vi "IMU.vi"(8 "error in (no error)":errorcluster, 11 "VISA Refnum in":refnum<visa-resource-name>) -> (0 "error out":errorcluster, 1 "Waveform Chart":cluster{"Yaw":dbl, "Pitch":dbl, "Roll":dbl}(graph), 2 "IMU Text":string, 3 "VISA Refnum out":refnum<visa-resource-name>, 5 "IMU Data Cluster":T1)   [LabVIEW 2016]
uses:
  Project Custom Controls/IMU Data Cluster.ctl
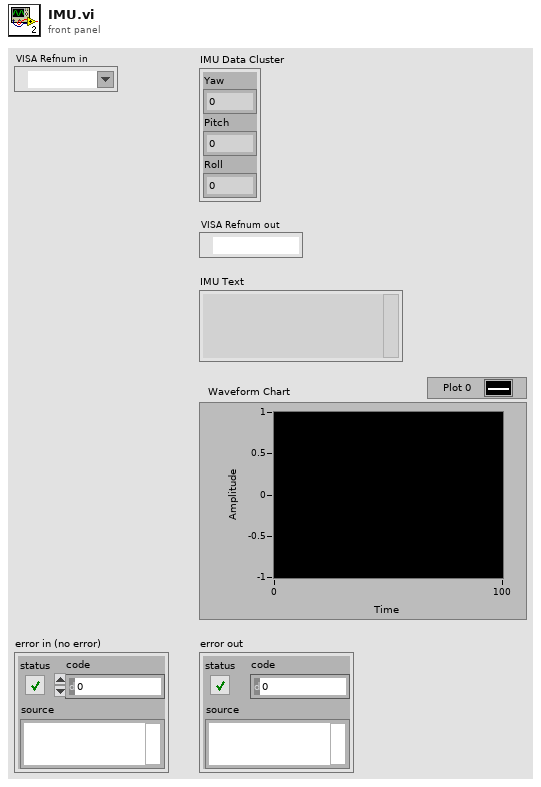
[diagram p1: front panel]
types:
  T1 = typedef "IMU Data Cluster.ctl" = cluster{"Yaw":dbl, "Pitch":dbl, "Roll":dbl}
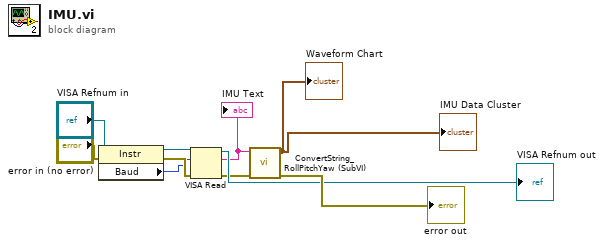
[diagram p0: block diagram]
diagram:
  n1 = property class="Instr"(reference="VISA Refnum in", error in="error in (no error)") -> (reference out=w3:refnum<visa-resource-name>, error out=w2:errorcluster, "Baud"=w1:u32)
  n2 = VISA Read(VISA resource name=w3, byte count=w1, error in (no error)=w2) -> (VISA resource name out=→"VISA Refnum out":refnum<visa-resource-name>, read buffer=w5:string, error out=w4:errorcluster)  [unwired: 1 out]
  "IMU Text" <- w5
  n3 = call "ConvertString_RollPitchYaw (SubVI).vi"("error in (no error)"=w4, "IMU String Data"=w5) -> ("error out"=→"error out":errorcluster, "IMU Data Cluster"=→"Waveform Chart" →"IMU Data Cluster":T1)  [unwired: 8 in]
